vi "ListAllFiles.vi"(5 "subFolders to Exclude":string[](array[string]), 7 "subfolder":bool, 8 "error in":errorcluster, 10 "pattern":string="*.vi", 11 "vi path":path) -> (0 "error out":errorcluster, 3 "All Files":path[](array[path]))   [LabVIEW 2011]
panel:
  out "size(s)":i32
  # "only if folder"
  # "if file: retunf file (pattern??)\nif folder retun all in folder \nif folder and subfolder=t return also subfolders"
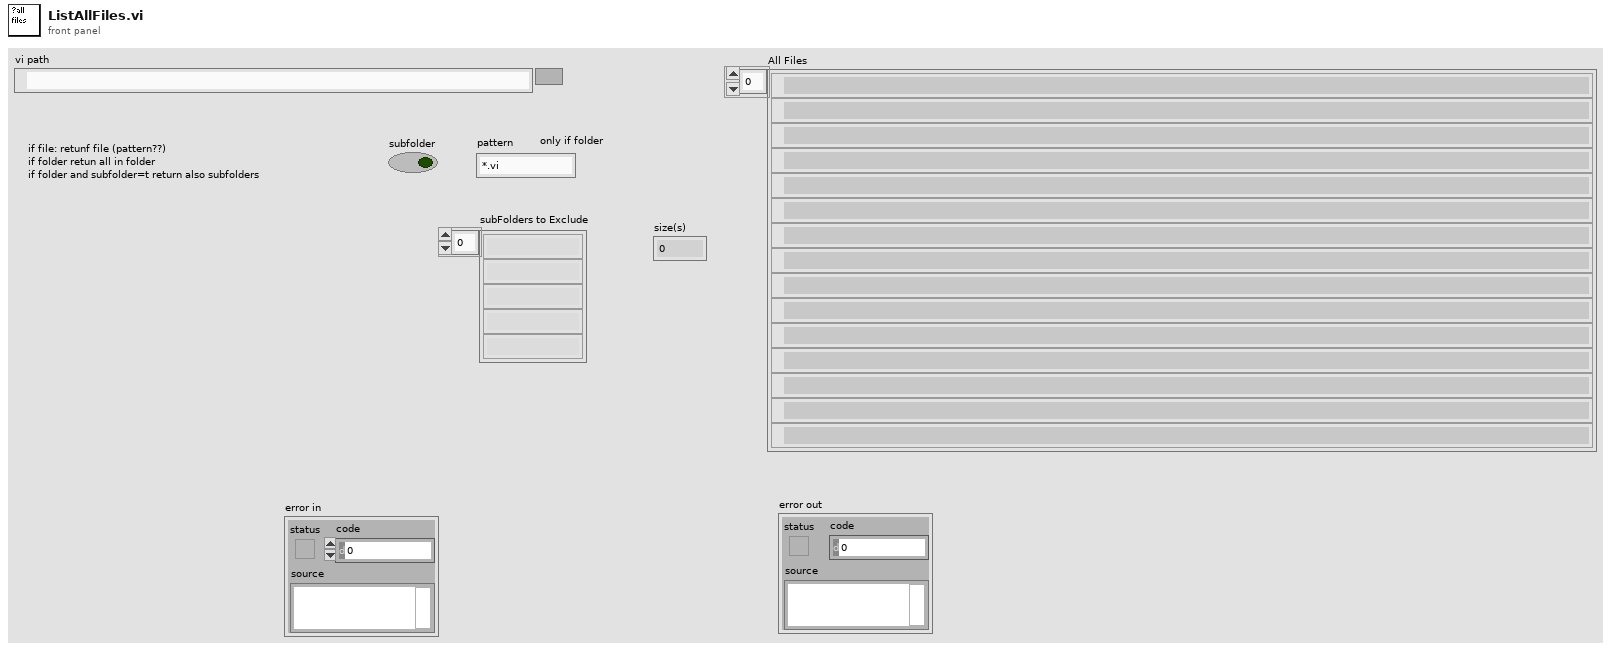
[diagram p1: front panel]
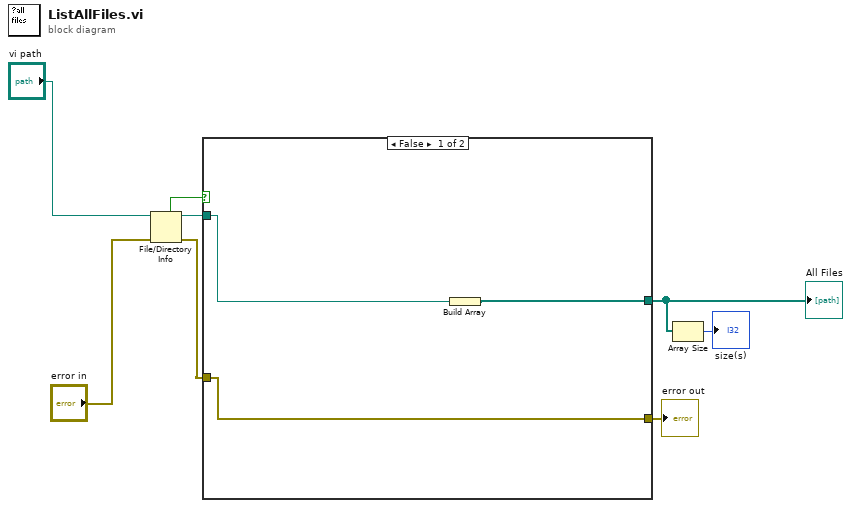
[diagram p0: block diagram]
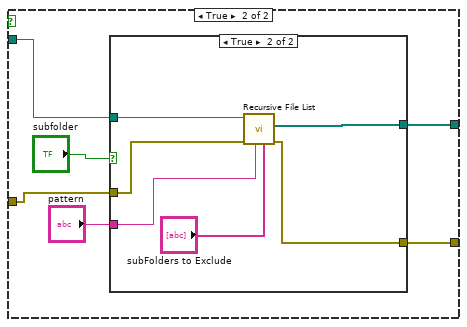
[diagram p2: hidden frame]
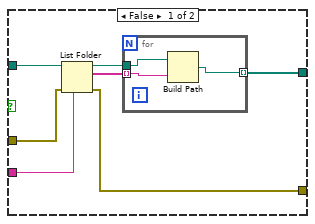
[diagram p3: hidden frame]
diagram:
  n1 = File/Directory Info(path="vi path", error in="error in") -> (path out=w6:path, directory=w7:bool, error out=w2:errorcluster)  [unwired: 4 out]
  n2 = case shown="False" w7 {
    tunnel: w6 -> [w11 w17]
    tunnel: [w10 w16] -> w5
    tunnel: [w9 w13] -> w3
    tunnel: w2 -> [w9 w12]
    frame False {
      n3 = Build Array(w11) -> (w10:path[])
    }
    frame True {
      n4 = case shown="True" "subfolder" {
        tunnel: w17 -> [w24 w33]
        tunnel: [w21 w31] -> w16
        tunnel: "pattern" -> [w20 w30]
        tunnel: [w19 w29] -> w13
        tunnel: w12 -> [w18 w28]
        frame False {
          n5 = List Folder(path=w24, pattern=w20, error in=w18) -> (path out=w23:path, filenames=w22:string[], error out=w19:errorcluster)  [unwired: 1 in, 1 out]
          n6 = for {
            tunnel: w23 -> [w27]
            tunnel: w22 -> [w26] mode=indexing
            tunnel: [w25] -> w21 mode=indexing
            n7 = Build Path(base path=w27, name or relative path=w26) -> (appended path=w25:path)
          }
        }
        frame True {
          n8 = call <vilib>:"Recursive File List.vi"("Folders to Exclude"="subFolders to Exclude", "pattern"=w30, "error in (no error)"=w28, "Folder Path"=w33) -> ("error out"=w29:errorcluster, "All Files in Dir"=w31:path[])  [unwired: 3 in, 3 out]
        }
      }
    }
  }
  "All Files" <- w5
  "error out" <- w3
  n9 = Array Size(array=w5) -> (size(s)=→"size(s)":i32)
